vi "dsdata.vi"() -> ()   [LabVIEW 2020]
doc: "This global variable contains data from the FMS system as well as the FRC 4265 Dashboard including safety overrides, calibration commands, and configuration parameters. These data are updated during all robot modes. Robot commands should never be placed in this global variable."
uses:
  <vilib>/Rock Robotics/WPI/DriverStation/WPI_DriverStationRobotMode2.ctl
panel:
  out "Running_Systems_Check":bool
  out "Driver_DPad":T1(ring)
  out "Test_Actuator_Period (s)":dbl
  out "Driver_Joystick_Calibrations":dbl[](array[numeric])
  out "Calibrate_Joysticks":bool
  out "Robot_is_Autonomous":bool
  out "Test_Actuator_Value":dbl
  out "Test_Actuator_Name":string
  out "Tune_Tab":bool
  out "Robot Mode":T2
  # "--FMS--"
  # "--driver joystick--"
  # "--overrides--"
  # "--tune tab--"
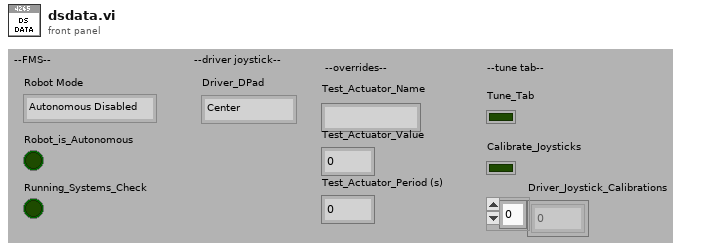
[diagram p1: front panel]
types:
  T1 = enum16{"Center", "North", "NorthWest", "West", "SouthWest", "South", "SouthEast", "East", "NorthEast"}
  T2 = typedef "WPI_DriverStationRobotMode2.ctl" = enum16{"Autonomous Disabled", "Autonomous Enabled", "Teleop Disabled", "Teleop Enabled", "Disconnected", "Finish", "Test Disabled", "Test Enabled", "Emergency Stopped"}
diagram:
